vi "LabVIEW 4 MiniGen_Basic.vi"(3 "error in (no error)":errorcluster, 5 "write buffer":string="r128") -> (0 "error out":errorcluster)   [LabVIEW 2020]
uses:
  <vilib>/Instr/_visa.llb/VISA Flush IO Buffer Mask.ctl
  <vilib>/Instr/_visa.llb/VISA Configure Serial Port (Instr).vi
panel:
  in  "VISA resource name":refnum<visa-resource-name>="COM5"
  out "read buffer":string="Frequency changed to 200.00\r\n"
  out "XY Graph":cluster{i32[], dbl[]}[](graph)=[{[0, 1, 2, 3, 4, 5, 6, 7, 8, 9, 10, 11, 12, 13, 14, 15, 16, 17, 18, 19, 20, 21, 22, 23, 24, 25, 26, 27, 28, 29, 30, 31, 32, 33, 34, 35, 36, 37, 38, 39, 40, 41, 42, 43, 44, 45, 46, 47, 48, 49, 50, 51, 52, 53, 54, 55, 56, 57, 58, 59, 60, 61, 62, 63, 64, 65, 66, 67, 68, 69, 70, 71, 72, 73, 74, 75, 76, 77, 78, 79, 80, 81, 82, 83, 84, 85, 86, 87, 88, 89, 90, 91, 92, 93, 94, 95, 96, 97, 98, 99, 100, 101, 102, 103, 104, 105, 106, 107, 108, 109, 110, 111, 112, 113, 114, 115, 116, 117, 118, 119, 120, 121, 122, 123, 124, 125, 126, 127], [2.177734375, 2.177734375, 2.16796875, 2.1533203125, 2.1240234375, 2.0849609375, 2.041015625, 1.9873046875, 1.9287109375, 1.865234375, 1.7919921875, 1.71875, 1.6455078125, 1.5673828125, 1.4990234375, 1.4306640625, 1.3671875, 1.30859375, 1.259765625, 1.2158203125, 1.181640625, 1.1572265625, 1.142578125, 1.142578125, 1.1474609375, 1.162109375, 1.19140625, 1.2255859375, 1.26953125, 1.3232421875, 1.3818359375, 1.4501953125, 1.5185546875, 1.5869140625, 1.6650390625, 1.73828125, 1.8115234375, 1.8798828125, 1.943359375, 2.001953125, 2.0556640625, 2.099609375, 2.1337890625, 2.158203125, 2.1728515625, 2.177734375, 2.177734375, 2.1630859375, 2.1435546875, 2.109375, 2.0703125, 2.021484375, 1.9677734375, 1.904296875, 1.8359375, 1.7626953125, 1.689453125, 1.6162109375, 1.54296875, 1.474609375, 1.40625, 1.3427734375, 1.2890625, 1.240234375, 1.201171875, 1.171875, 1.15234375, 1.1376953125, 1.1376953125, 1.15234375, 1.171875, 1.201171875, 1.240234375, 1.2841796875, 1.3427734375, 1.4013671875, 1.4697265625, 1.5380859375, 1.6162109375, 1.689453125, 1.7626953125, 1.8359375, 1.8994140625, 1.962890625, 2.021484375, 2.0703125, 2.109375, 2.138671875, 2.1630859375, 2.1728515625, 2.177734375, 2.1728515625, 2.1533203125, 2.12890625, 2.0947265625, 2.0556640625, 2.001953125, 1.943359375, 1.8798828125, 1.8115234375, 1.73828125, 1.6650390625, 1.591796875, 1.5185546875, 1.4501953125, 1.3818359375, 1.3232421875, 1.26953125, 1.2255859375, 1.19140625, 1.162109375, 1.1474609375, 1.1376953125, 1.142578125, 1.1572265625, 1.181640625, 1.2109375, 1.2548828125, 1.30859375, 1.3623046875, 1.42578125, 1.494140625, 1.5673828125, 1.640625, 1.7138671875, 1.787109375, 1.8603515625, 1.923828125]}]
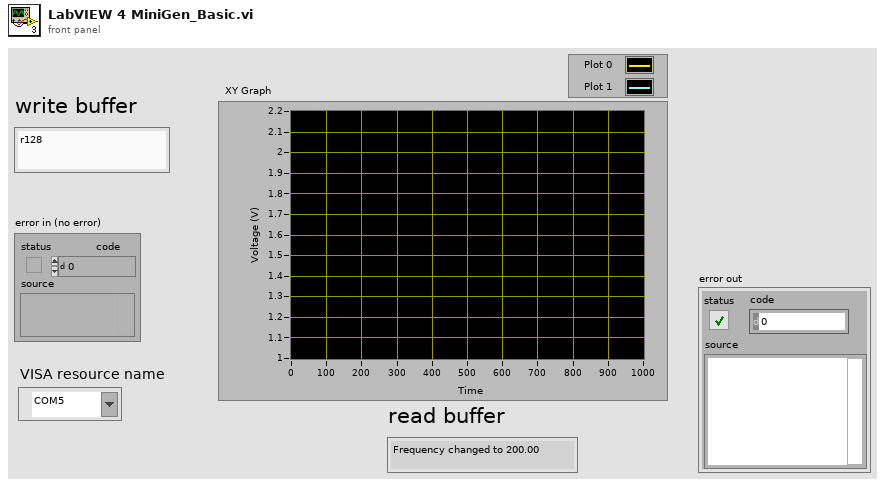
[diagram p1: front panel]
types:
  T1 = typedef "VISA Flush IO Buffer Mask.ctl" = u16
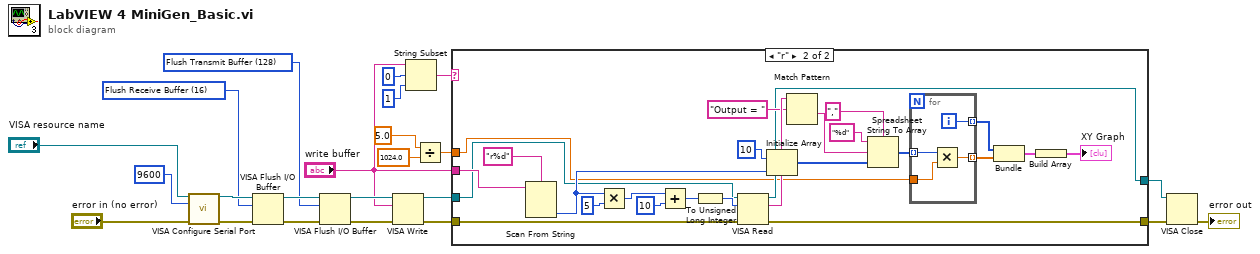
[diagram p0: block diagram]
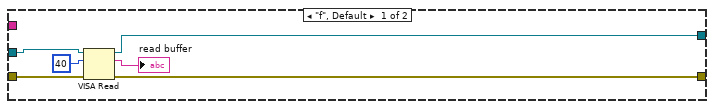
[diagram p2: hidden frame]
diagram:
  w17 = T1 128 items=["Flush Receive Buffer"=16, "Write Transmit Buffer to Device"=32, "Flush Receive Buffer (No I/O)"=64, "Flush Transmit Buffer"=128] ("Mask")
  w20 = T1 16 items=["Flush Receive Buffer"=16, "Write Transmit Buffer to Device"=32, "Flush Receive Buffer (No I/O)"=64, "Flush Transmit Buffer"=128] ("Mask")
  n1 = call-poly "VISA Configure Serial Port"("VISA resource name"="VISA resource name", "baud rate (9600)"=u32 9600, "error in (no error)"="error in (no error)") -> ("VISA resource name out"=w22:refnum<visa-resource-name>, "error out"=w21:errorcluster)  [unwired: 11 in]
  n2 = VISA Flush I/O Buffer(VISA resource name=w22, mask (16)=w20, error in (no error)=w21) -> (VISA resource name out=w19:refnum<visa-resource-name>, error out=w18:errorcluster)
  n3 = VISA Flush I/O Buffer(VISA resource name=w19, mask (16)=w17, error in (no error)=w18) -> (VISA resource name out=w16:refnum<visa-resource-name>, error out=w15:errorcluster)
  n4 = VISA Write(VISA resource name=w16, write buffer="write buffer", error in (no error)=w15) -> (VISA resource name out=w11:refnum<visa-resource-name>, error out=w10:errorcluster)  [unwired: 1 out]
  n5 = String Subset(string="write buffer", offset (0)=0, length (rest)=1 ("length (rest)")) -> (substring=w6:string)
  n6 = Divide(x=5.0, y=1024.0) -> (x/y=w1:dbl)
  n7 = case shown="\"r\"" w6 {
    tunnel: [w28 w31] -> w14
    tunnel: [w25 w32] -> w13
    tunnel: w11 -> [w27 w34]
    tunnel: w10 -> [w29 w33]
    tunnel: "write buffer" -> [_ w54]
    tunnel: w1 -> [_ w30]
    frame "f", Default {
      n8 = VISA Read(VISA resource name=w27, byte count=u32 40, error in (no error)=w29) -> (VISA resource name out=w25:refnum<visa-resource-name>, read buffer=→"read buffer":string, error out=w28:errorcluster)  [unwired: 1 out]
    }
    frame "r" {
      n9 = Scan From String(format string="r%d", input string=w54) -> (output 1=w41:i32)  [unwired: 3 in, 3 out]
      n10 = Multiply(x=w41, y=5) -> (x*y=w51:i32)
      n11 = Add(x=w51, y=10) -> (x+y=w49:i32)
      n12 = To Unsigned Long Integer(number=w49) -> (unsigned 32bit integer=w48:u32)
      n13 = VISA Read(VISA resource name=w34, byte count=w48, error in (no error)=w33) -> (VISA resource name out=w32:refnum<visa-resource-name>, read buffer=w47:string, error out=w31:errorcluster)  [unwired: 1 out]
      n14 = Initialize Array(10 ("y"), w41) -> (w40:i32[])
      n15 = Match Pattern(string=w47, regular expression="Output = ") -> (after substring=w45:string)  [unwired: 1 in, 3 out]
      n16 = Spreadsheet String To Array(delimiter (Tab)=",", format string="%d", spreadsheet string=w45, array type (2D Dbl)=w40) -> (array=w39:i32[])
      n17 = for {
        tunnel: w39 -> [w57] mode=indexing
        tunnel: [w55] -> w37 mode=indexing
        tunnel: [w58] -> w38 mode=indexing
        tunnel: w30 -> [w56]
        i -> [w58]
        n18 = Multiply(x=w57, y=w56) -> (x*y=w55:dbl)
      }
      n19 = Bundle(w38, w37) -> (w36:cluster{i32[], dbl[]})  [unwired: 1 in]
      n20 = Build Array(w36) -> (→"XY Graph":cluster{i32[], dbl[]}[])
    }
  }
  n21 = VISA Close(VISA resource name=w13, error in (no error)=w14) -> (error out=→"error out":errorcluster)
